vi "NarrowOscilattions1.vi"(1 "Max Angle":dbl, 2 "Angle":dbl, 3 "dY2":dbl, 4 "dX2":dbl, 5 "dY1":dbl, 6 "dX1":dbl) -> (0 "Backward Displacement!":bool)   [LabVIEW 2017]
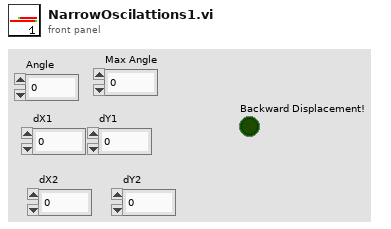
[diagram p1: front panel]
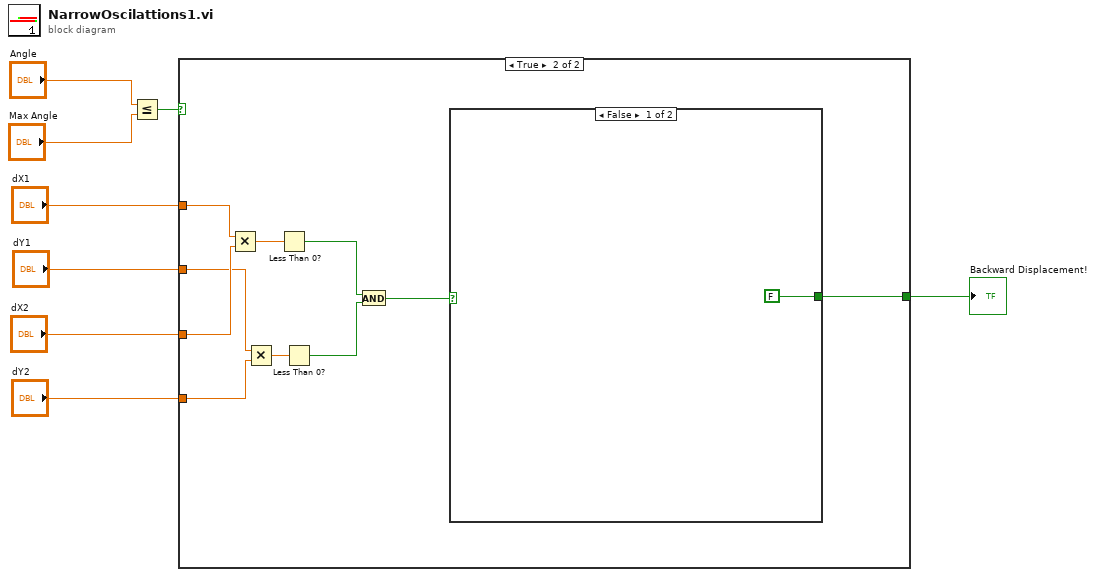
[diagram p0: block diagram]
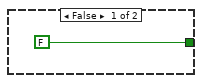
[diagram p2: hidden frame]
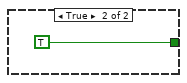
[diagram p3: hidden frame]
diagram:
  n1 = Less Or Equal?(x="Angle", y="Max Angle") -> (x <= y?=w6:bool)
  n2 = case shown="True" w6 {
    tunnel: "dX1" -> [_ w19]
    tunnel: "dY1" -> [_ w17]
    tunnel: "dX2" -> [_ w18]
    tunnel: "dY2" -> [_ w16]
    tunnel: [FALSE w10] -> w1
    frame False {
    }
    frame True {
      n3 = Multiply(x=w19, y=w18) -> (x*y=w15:dbl)
      n4 = Multiply(x=w17, y=w16) -> (x*y=w14:dbl)
      n5 = Less Than 0?(x=w15) -> (x < 0?=w13:bool)
      n6 = Less Than 0?(x=w14) -> (x < 0?=w12:bool)
      n7 = And(x=w13, y=w12) -> (x .and. y?=w11:bool)
      n8 = case shown="False" w11 {
        tunnel: [FALSE TRUE] -> w10
        frame False {
        }
        frame True {
        }
      }
    }
  }
  "Backward Displacement!" <- w1
